vi "3-13-shui xian hua.vi"() -> ()   [LabVIEW 2018]
panel:
  out "数组":i32[](array[numeric])
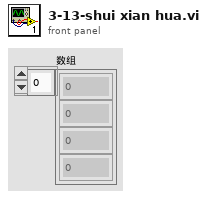
[diagram p1: front panel]
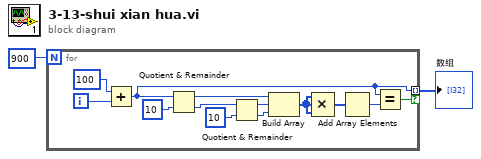
[diagram p0: block diagram]
diagram:
  n1 = for {
    N: 900 -> [_]
    tunnel: [w4] -> w1 mode=indexing if=w3
    i -> [w15]
    n2 = Add(x=100, y=w15) -> (x+y=w4:i32)
    n3 = Quotient & Remainder(x=w4, y=10) -> (x-y*floor(x/y)=w8:i32, floor(x/y)=w11:i32)
    n4 = Quotient & Remainder(x=w11, y=10) -> (x-y*floor(x/y)=w9:i32, floor(x/y)=w10:i32)
    n5 = Build Array(w8, w9, w10) -> (w7:i32[])
    n6 = Compound Arithmetic op=MULTIPLY(w7, w7, w7) -> (w6:i32[])
    n7 = Add Array Elements(numeric array=w6) -> (sum=w5:i32)
    n8 = Equal?(x=w4, y=w5) -> (x = y?=w3:bool)
  }
  "数组" <- w1
